vi "Open Device.vi"(0 "USRP RIO device":T1="RIO0", 11 "error in":errorcluster) -> (4 "niUsrpRio Session (out)":T2={"Global Settings Register Bus"=refnum, "Radio 0 Settings Register Bus"=refnum, "Rx NI-USRP session"="", "Tx NI-USRP session"="", "FPGA Interface"=refnum, "RIO Interface Number"=0, "EEPROM Header"={"Checksum"=0, "Product Code"=0, "Hardware Current Version"=0, "Hardware Oldest Compatible Version"=0, "EEPROM Map Current Version"=0, "EEPROM Map Oldest Compatible Version"=0, "User Password"="", "Pointer to Factory Header"=0, "Pointer to User Header"=0, "Recommended Interval"=0, "Number of Reserved Bytes"=9, "Number of Daughterboards"=0, "Daughterboard IDs"=[], "Daughterboard Serial Numbers"=[]}, "Device Data Header"={"Checksum"=0, "Number of Channels"=0, "Number of Gain Settings"=[], "Pointer to Characterization Data"=[], "Number of Reserved Bytes"=27, "Number of Frequencies"=[]}, "EEPROM Characterization Header"={"Checksum"=0, "Date"=timestamp(0 s since 1904-01-01), "Temperature"=0.0, "Misc. Info"="", "Pointer to Device Data Header"=0, "Number of Reserved Bytes"=28}, "Characterization Data"=[], "Characterization Data Valid?"=FALSE, "Radio 1 Settings Register Bus"=refnum, "Radio Settings Bus Semaphore"=refnum} {"Characterization Data"."Frequencies [Hz]" format="%#_6p"; "EEPROM Characterization Header"."Pointer to Device Data Header" format="%x"; "EEPROM Characterization Header"."Checksum" format="%x"; "Device Data Header"."Pointer to Characterization Data" format="%x"; "Device Data Header"."Checksum" format="%x"; "EEPROM Header"."Pointer to User Header" format="%x"; "EEPROM Header"."Pointer to Factory Header" format="%x"; "EEPROM Header"."Product Code" format="%x"; "EEPROM Header"."Checksum" format="%x"}, 15 "error out":errorcluster)   [LabVIEW 2013]
doc: "Opens a session to the USRP RIO design library. Creates the necessary connections to the hardware and initializes the device.\n\n<B>Input Parameters</B>\n\n<B>USRP RIO device</B> is the specific device to open a session to.\n\n<B>error in</B> describes error conditions that occur before this node runs. This input provides standard 'error in' functionality.\n\n<B>Output Parameters</B>\n\n<B>niUsrpRio Session (out)</B> is a new niUsrpRio session used in all subsequent USRP RIO design library host VIs.\n\n<B>error out</B> contains error information. This output provides standard 'error out' functionality."
uses:
  <instrlib>/niUsrpRio/Config/v1/Host/Public/niUsrpRio Session.ctl
  <instrlib>/_niInstr/Register Bus/v0/Host/Public/Register Bus Session.ctl
  <instrlib>/_niInstr/Register Bus/v0/Host/Private/Session Data.ctl
  <instrlib>/niUsrpRio/Config/v1/Host/Public/EEPROM Header.ctl
  <instrlib>/niUsrpRio/Config/v1/Host/Public/EEPROM Device Data Header.ctl
  <instrlib>/niUsrpRio/Config/v1/Host/Public/EEPROM Characterization Header.ctl
  <instrlib>/niUsrpRio/Config/v1/Host/Public/Characterization Data.ctl
  <instrlib>/niUsrpRio/Config/v1/Host/Public/IQ Imbalance.ctl
  <vilib>/userdefined/Silver/nirio_resource_slv.ctl
  <instrlib>/niUsrpRio/Config/v1/Host/niUsrpRio Config v1 Host.lvlib
  <instrlib>/_niInstr/Register Bus/v0/Host/niInstr Register Bus v0 Host.lvlib
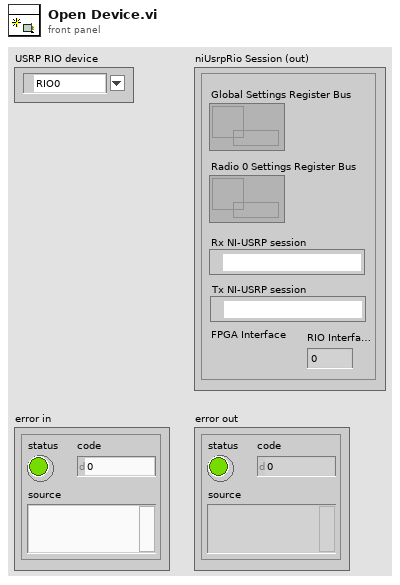
[diagram p1: front panel]
types:
  T1 = typedef "nirio_resource_slv.ctl" = tag
  T2 = typedef "niUsrpRio Config v1 Host.lvlib/niUsrpRio Session.ctl" = cluster{"Global Settings Register Bus":T3, "Radio 0 Settings Register Bus":T3, "Rx NI-USRP session":refnum<k15>, "Tx NI-USRP session":refnum<k15>, "FPGA Interface":refnum<k20>, "RIO Interface Number":u32, "EEPROM Header":T4, "Device Data Header":T5, "EEPROM Characterization Header":T6, "Characterization Data":T7[], "Characterization Data Valid?":bool, "Radio 1 Settings Register Bus":T3, "Radio Settings Bus Semaphore":T9}
  T3 = typedef "niInstr Register Bus v0 Host.lvlib/Register Bus Session.ctl" = refnum<queue>
  T4 = typedef "niUsrpRio Config v1 Host.lvlib/EEPROM Header.ctl" = cluster{"Checksum":u32, "Product Code":u16, "Hardware Current Version":u16, "Hardware Oldest Compatible Version":u16, "EEPROM Map Current Version":u16, "EEPROM Map Oldest Compatible Version":u16, "User Password":string, "Pointer to Factory Header":u32, "Pointer to User Header":u32, "Recommended Interval":u16, "Number of Reserved Bytes":i32, "Number of Daughterboards":u8, "Daughterboard IDs":u16[], "Daughterboard Serial Numbers":string[]}
  T5 = typedef "niUsrpRio Config v1 Host.lvlib/EEPROM Device Data Header.ctl" = cluster{"Checksum":u32, "Number of Channels":u8, "Number of Gain Settings":u16[], "Pointer to Characterization Data":u32[], "Number of Reserved Bytes":i32, "Number of Frequencies":u16[]}
  T6 = typedef "niUsrpRio Config v1 Host.lvlib/EEPROM Characterization Header.ctl" = cluster{"Checksum":u32, "Date":timestamp, "Temperature":sgl, "Misc. Info":string, "Pointer to Device Data Header":u32, "Number of Reserved Bytes":i32}
  T7 = typedef "niUsrpRio Config v1 Host.lvlib/Characterization Data.ctl" = cluster{"Gains[dB]":dbl[], "Frequencies [Hz]":dbl[], "IQ Imbalance Table":T8[], "Measured Gains[dB]":dbl[][]}
  T8 = typedef "niUsrpRio Config v1 Host.lvlib/IQ Imbalance.ctl" = cluster{"Gain Imbalance [linear]":dbl, "Phase Imbalance [radians]":dbl, "Offset":cdb}
  T9 = typedef "Semaphore RefNum" = refnum<k1>
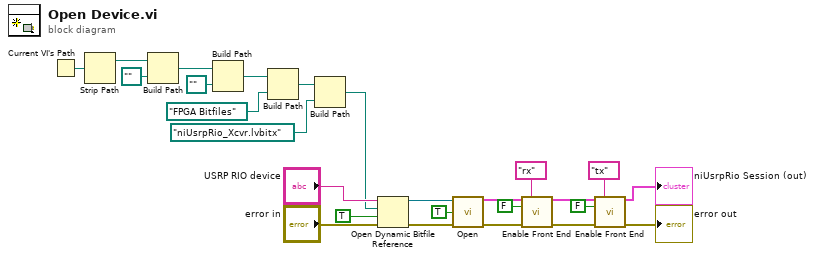
[diagram p0: block diagram]
diagram:
  n1 = Current VI's Path() -> (path=w25:path)
  n2 = Strip Path(path=w25) -> (stripped path=w24:path)  [unwired: 1 out]
  n3 = Build Path(base path=w24, name or relative path=path "..") -> (appended path=w14:path)
  n4 = Build Path(base path=w14, name or relative path=path "..") -> (appended path=w13:path)
  n5 = Build Path(base path=w13, name or relative path=path "FPGA Bitfiles") -> (appended path=w20:path)
  n6 = Build Path(base path=w20, name or relative path=path "niUsrpRio_Xcvr.lvbitx") -> (appended path=w11:path)
  n7 = Open Dynamic Bitfile Reference(0:"USRP RIO device", 1:w11, 2:TRUE ("Run When Loaded"), 3:"error in") -> (5:w19:refnum<k20>, 8:w18:errorcluster)  [unwired: 1 in]
  n8 = call <instrlib>:"Open.vi"("fpga ref"=w19, "reset?"=TRUE, "Error In"=w18) -> ("niUsrpRio Session (out)"=w4:T2, "Error Out"=w10:errorcluster)  [unwired: 11 in]
  n9 = call <instrlib>:"Enable Front End.vi"("niUsrpRio Session"=w4, "scope"="rx", "enable"=FALSE, "error in"=w10) -> ("niUsrpRio Session (out)"=w5:T2, "error out"=w9:errorcluster)  [unwired: 10 in]
  n10 = call <instrlib>:"Enable Front End.vi"("niUsrpRio Session"=w5, "scope"="tx", "enable"=FALSE, "error in"=w9) -> ("niUsrpRio Session (out)"=→"niUsrpRio Session (out)":T2, "error out"=→"error out":errorcluster)  [unwired: 10 in]
